vi "Hatch Panel Reset.vi"(0 "InnerRefnum":string, 1 "OuterRefnum":string, 2 "DriveRefnum":string, 3 "HatchReset?":bool) -> ()   [LabVIEW 2018]
uses:
  <vilib>/Rock Robotics/WPI/Solenoid/WPI_SolenoidValue.ctl
  <vilib>/Rock Robotics/WPI/Utilities/WPI_GetSetVariantRefNum.vi
  <vilib>/Rock Robotics/WPI/RobotDrive/WPI_RobotDriveArcadeDrive_Standard(NoSaturation).vi
  <vilib>/Rock Robotics/WPI/Solenoid/WPI_SolenoidSetEnum.vi
  Robot Global Data.vi
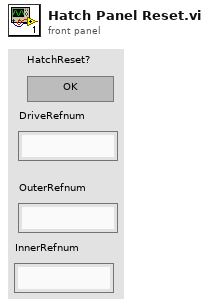
[diagram p1: front panel]
types:
  T1 = typedef "WPI_SolenoidValue.ctl" = enum16{"Off", "On", "Forward", "Reverse"}
  T2 = typedef "WPI_RobotDriveDevRef.ctl" = cluster{"DevStatus":errorcluster, "Motors[]":T3[], "Square Inputs":bool, "Max Output":dbl}
  T3 = typedef "WPI_MotorControlDeviceRef.ctl" = cluster{"DeviceStatus":errorcluster, "Type":T4, "PWM":cluster{"PWM Channel":T5, "DeadBand":T6}, "CAN":cluster{"Device Number":u8, "SetOutput VI Ref":variant, "GetOutput VI Ref":variant, "Enable VI Ref":variant, "Disable VI Ref":variant, "Data":variant}, "Invert":bool, "DIO PWM":cluster{"PWM \"Enable\" Channel":T5, "DIOChannel":T7, "PWM Rate":dbl}}
  T4 = typedef "WPI_MotorControlType.ctl" = enum16{"PWM", "CAN", "DIO PWM"}
  T5 = typedef "FPGA_DIOPWMChannel.ctl" = enum8{"PWM 0", "PWM 1", "PWM 2", "PWM 3", "PWM 4", "PWM 5", "PWM 6", "PWM 7", "PWM 8", "PWM 9", "PWM MXP 0", "PWM MXP 1", "PWM MXP 2", "PWM MXP 3", "PWM MXP 4", "PWM MXP 5", "PWM MXP 6", "PWM MXP 7", "PWM MXP 8", "PWM MXP 9", "Invalid"}
  T6 = typedef "WPI_PWMDeadband.ctl" = cluster{"Name":string, "maxPositivePwm":i32, "minPositivePwm":i32, "centerPwm":i32, "maxNegativePwm":i32, "minNegativePwm":i32, "angularRange":u16}
  T7 = typedef "FPGA_DIOChannel.ctl" = enum8{"DIO 0", "DIO 1", "DIO 2", "DIO 3", "DIO 4", "DIO 5", "DIO 6", "DIO 7", "DIO 8", "DIO 9", "DIO MXP 0", "DIO MXP 1", "DIO MXP 2", "DIO MXP 3", "DIO MXP 4", "DIO MXP 5", "DIO MXP 6", "DIO MXP 7", "DIO MXP 8", "DIO MXP 9", "DIO MXP 10", "DIO MXP 11", "DIO MXP 12", "DIO MXP 13", "DIO MXP 14", "DIO MXP 15", "SPI Port CS1", "SPI Port CS2", "SPI Port CS3", "SPI Port MISO", "SPI Port MOSI", "Invalid"}
  T8 = typedef "WPI_SolenoidDevRef.ctl" = cluster{"DevStatus":errorcluster, "Pneumatics Control Module":u8, "Forward Solenoid Channel":T9, "Reverse Solenoid Channel":T9}
  T9 = typedef "WPI_SolenoidChannel.ctl" = enum8{"Solenoid 0", "Solenoid 1", "Solenoid 2", "Solenoid 3", "Solenoid 4", "Solenoid 5", "Solenoid 6", "Solenoid 7", "Invalid"}
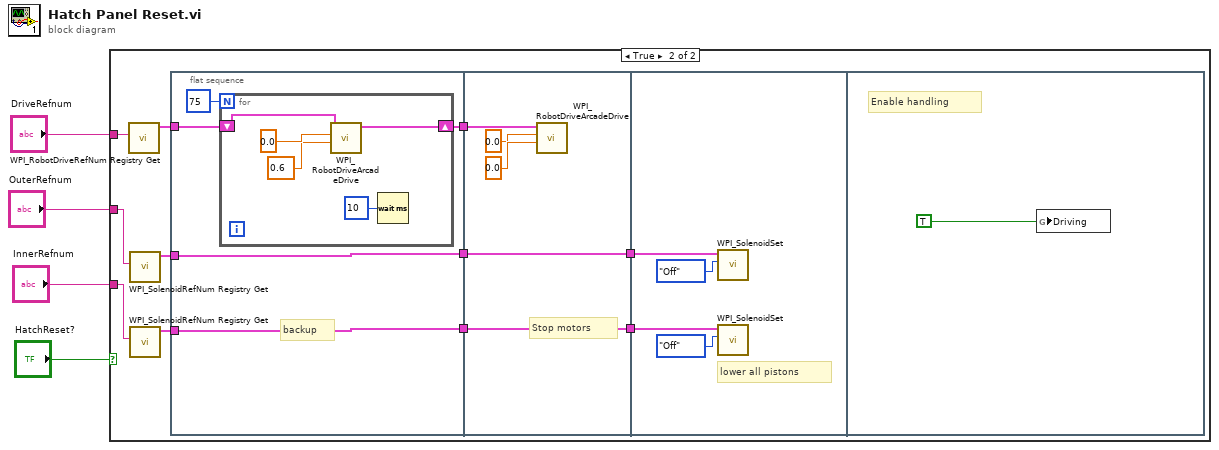
[diagram p0: block diagram]
diagram:
  n1 = case shown="True" "HatchReset?" {
    tunnel: "DriveRefnum" -> [_ w15]
    tunnel: "OuterRefnum" -> [_ w6]
    tunnel: "InnerRefnum" -> [_ w5]
    frame False {
    }
    frame True {
      n2 = call <vilib>:"WPI_RobotDriveRefNum Registry Get.vi"("refnum name"=w15) -> ("RobotDriveDevRef"=w14:T2)  [unwired: 9 in, 1 out]
      n3 = call <vilib>:"WPI_SolenoidRefNum Registry Get.vi"("refnum name"=w6) -> ("SolenoidDevRef"=w10:T8)  [unwired: 9 in, 1 out]
      n4 = call <vilib>:"WPI_SolenoidRefNum Registry Get.vi"("refnum name"=w5) -> ("SolenoidDevRef"=w7:T8)  [unwired: 9 in, 1 out]
      n5 = flat-sequence {
        tunnel: [w20] -> w13
        tunnel: [w19] -> w11
        tunnel: [w18] -> w8
        tunnel: w7 -> [w18]
        tunnel: w10 -> [w19]
        tunnel: w14 -> [w17]
        tunnel: w13 -> [w28]
        tunnel: [w27] -> w12
        tunnel: w11 -> [w27]
        tunnel: [w26] -> w9
        tunnel: w8 -> [w26]
        tunnel: w12 -> [w32]
        tunnel: w9 -> [w31]
        frame #0 {
          # "backup"
          n6 = for {
            N: 75 -> [_]
            shift-right: [w25] -> w20
            shift-left: w17 -> [w24]
            n7 = call-poly <vilib>:"WPI_RobotDriveArcadeDrive.vi"("Y axis value"=0.6, "X axis value"=0.0, "RobotDriveDevRef"=w24) -> ("RobotDriveDevRef"=w25:T2)  [unwired: 6 in, 2 out]
            n8 = Wait (ms)(milliseconds to wait=u32 10) -> ()  [unwired: 1 out]
          }
        }
        frame #1 {
          # "Stop motors"
          n9 = call-poly <vilib>:"WPI_RobotDriveArcadeDrive.vi"("Y axis value"=0.0, "X axis value"=0.0, "RobotDriveDevRef"=w28) -> ()  [unwired: 6 in, 3 out]
        }
        frame #2 {
          # "lower all pistons"
          n10 = call-poly <vilib>:"WPI_SolenoidSet.vi"("Value"=WPI_SolenoidValue."Off", "SolenoidDevRef"=w32) -> ()  [unwired: 8 in, 2 out]
          n11 = call-poly <vilib>:"WPI_SolenoidSet.vi"("Value"=WPI_SolenoidValue."Off", "SolenoidDevRef"=w31) -> ()  [unwired: 8 in, 2 out]
        }
        frame #3 {
          # "Enable handling"
          n12 = global write "Robot Global Data.vi" "Driving"(TRUE) -> ()
        }
      }
    }
  }
